vi "HomeVI.vi"() -> ()   [LabVIEW 2015]
uses:
  <vilib>/LabVIEW Interface for Arduino/Type Defs/Board Type.ctl
  <vilib>/express/express arith-compare/Formula/XNode/ExpressFormulaBlockNode.xnode
  <vilib>/LabVIEW Interface for Arduino/LabVIEW Interface for Arduino.lvlib
panel:
  in  "Tab Control":T1(tab)
  in  "Recipient's Name":string="DDU Smart Home"
  in  "Recipient's Email Address":string="ddusmarthome@gmail.com"
  in  "Arduino Mega COM Port":refnum<visa-resource-name>
  out "H_Current Mode":string
  in  "H_Mode Selector":enum32{"Automatic", "Manual"}(radio)
  in  "H_Light - Left":bool
  in  "H_Light - Right":bool
  in  "H_Fan Speed Regulator (% Percentage)":dbl(knob) scale=0.0..100.0
  out "H_Fan Speed ( % Percentage)":dbl(knob) scale=0.0..100.0
  out "H_Light - Left":bool
  out "H_Light - Right":bool
  out "H_Room Temprature":dbl(knob) scale=0.0..100.0
  out "H_Time":string
  out "K_Smoke":bool
  out "K_Light":bool
  in  "K_Mode Selector":enum32{"Automatic", "Manual"}(radio)
  out "K_Current Mode":string
  in  "K_Buzzer":bool
  in  "K_Light":bool
  out "K_Time":string
  out "B_Light":bool
  in  "B_Mode Selector":enum32{"Automatic", "Manual"}(radio)
  out "B_Current Mode":string
  in  "B_Light":bool
  out "B_Time":string
  in  "W_Light":bool
  out "W_Current Mode":string
  in  "W_Mode Selector":enum32{"Automatic", "Manual"}(radio)
  out "W_Light":bool
  out "W_Shower_Indicator":bool
  in  "Stop Button":bool
  in  "W_Mode Selector":enum32{"Automatic", "Manual"}(radio)
  out "W_Current Mode":string
  in  "W_Shower Switch":bool
  out "W_Time":string
  out "Last Intruder's Image":T2(plugin-control)
  # "Project Created By : \n                                     Patel Parth J. ( IC - 46 )\n                                     Patel Sarav M. (IC - 47)\n                                     Rai Aakash V. ( IC - 49 ) \n                                     Rupapara Pritesh N. ( IC - 51 )\n                                     Shah Vivek K. ( IC - 57 )"
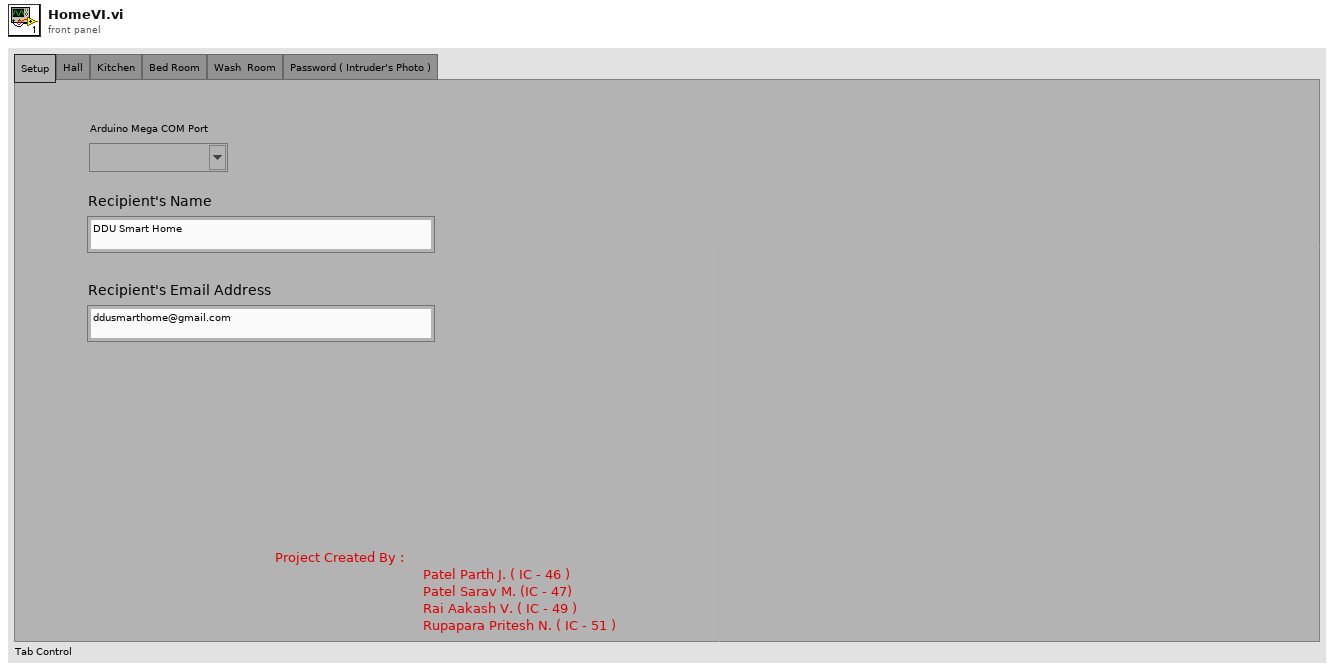
[diagram p1: front panel]
types:
  T1 = enum32{"Setup", "Hall", "Kitchen", "Bed Room", "Wash  Room", "Password ( Intruder's Photo )"}
  T2 = typedef "IMAQ Image.ctl" = refnum<image>
  T3 = typedef "LabVIEW Interface for Arduino.lvlib/Board Type.ctl" = enum16{"Uno", "Dimuelanove w/Atmega 328", "Mega 2560"}
  T4 = typedef "LabVIEW Interface for Arduino.lvlib/Arduino Resource.ctl" = cluster{"VISA resource":refnum<visa-resource-name>, "Board Type":T3, "Connection Type":enum8{"USB / Serial"}, "Bytes Per Packet (15)":u8}
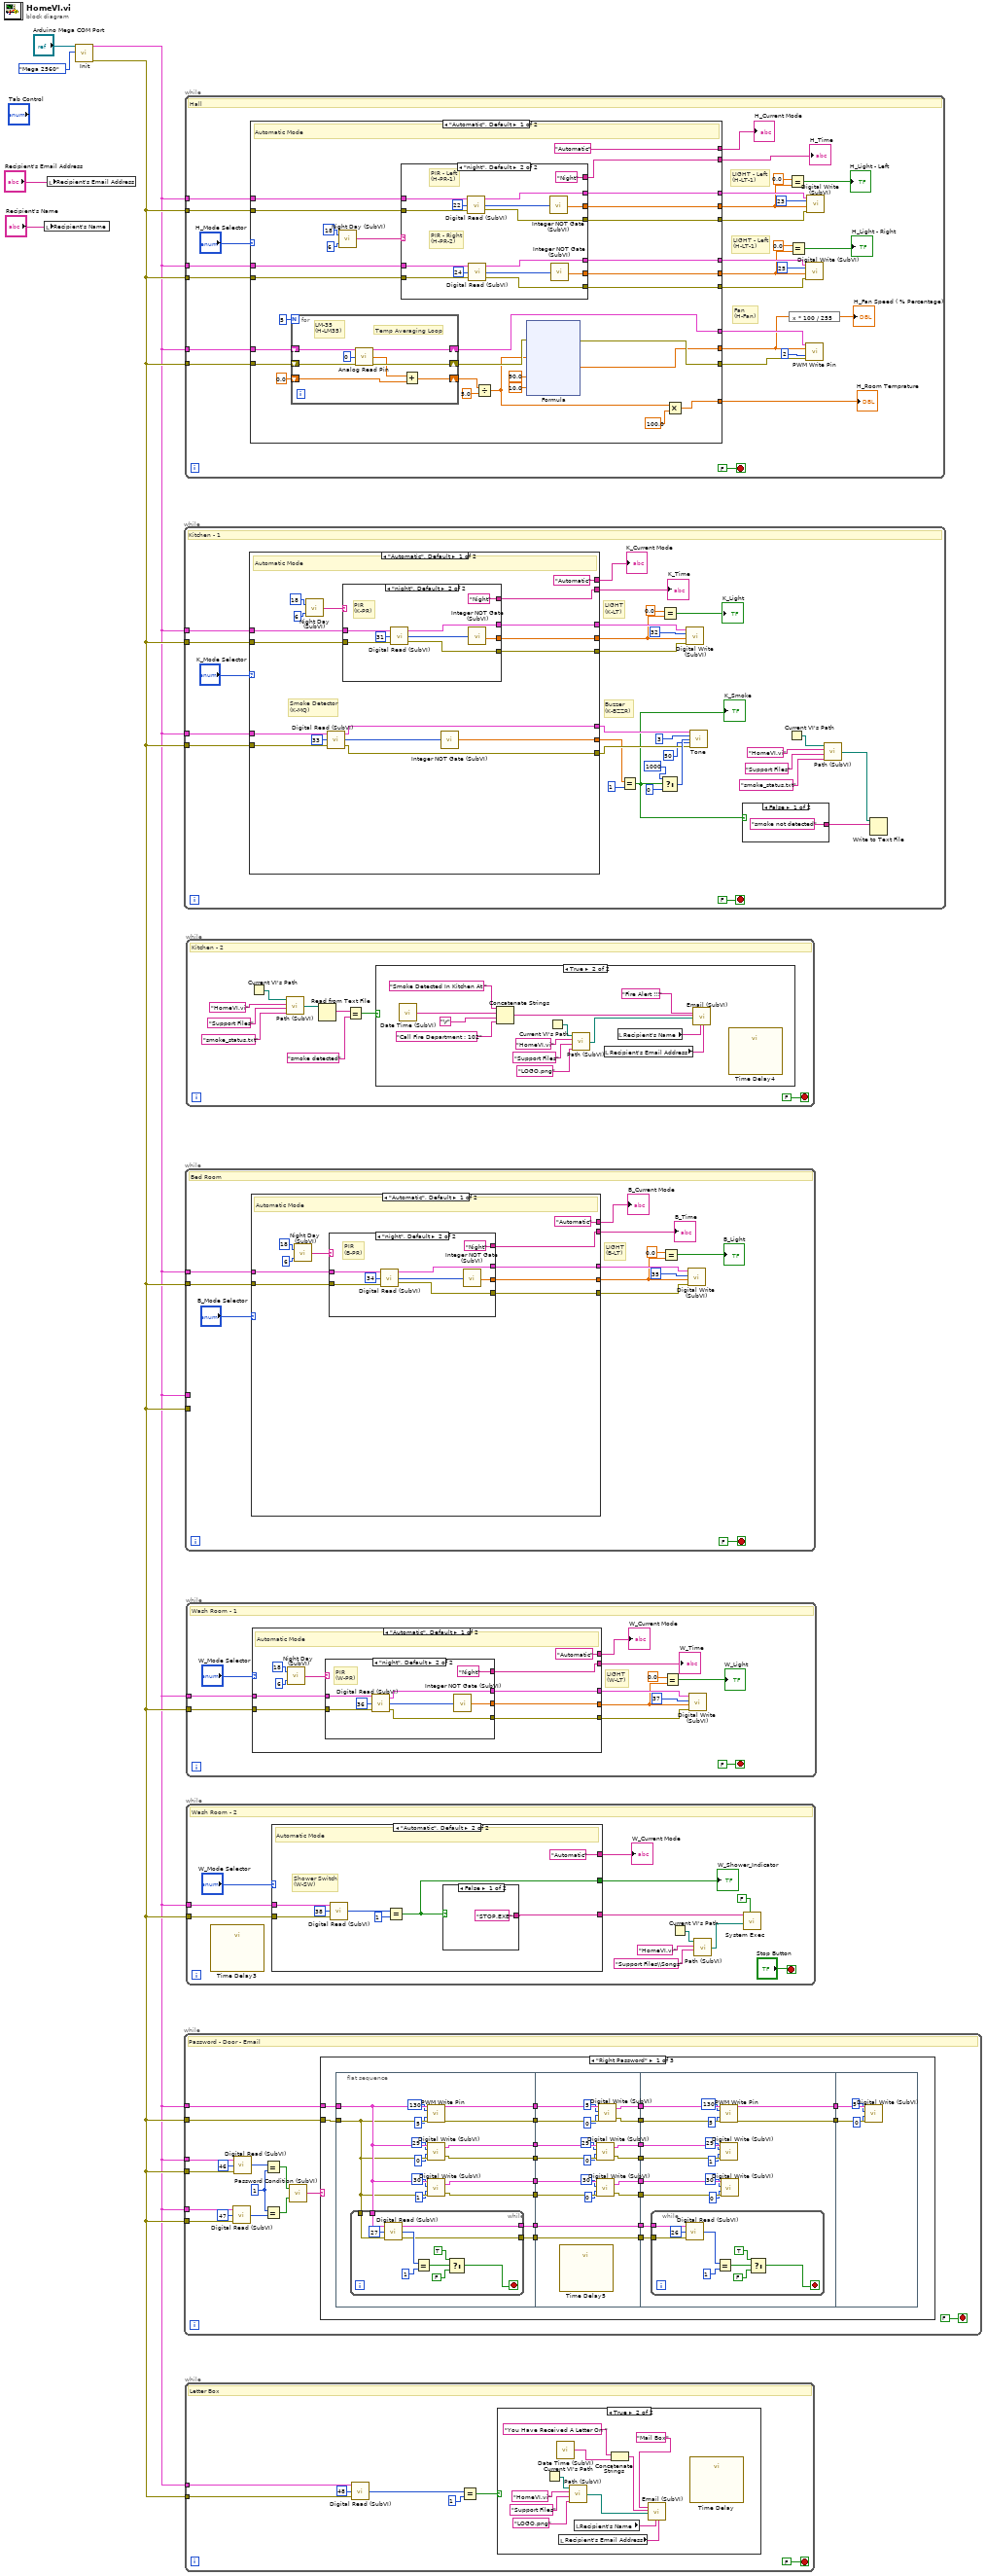
[diagram p0: block diagram]
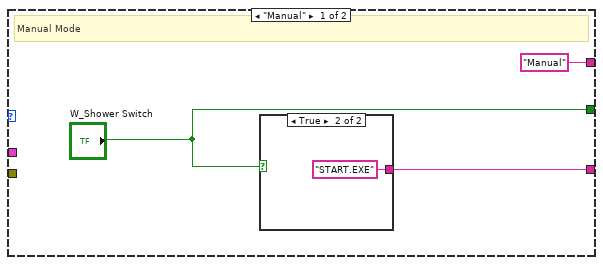
[diagram p4: hidden frame]
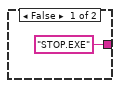
[diagram p5: hidden frame]
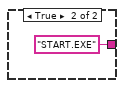
[diagram p6: hidden frame]
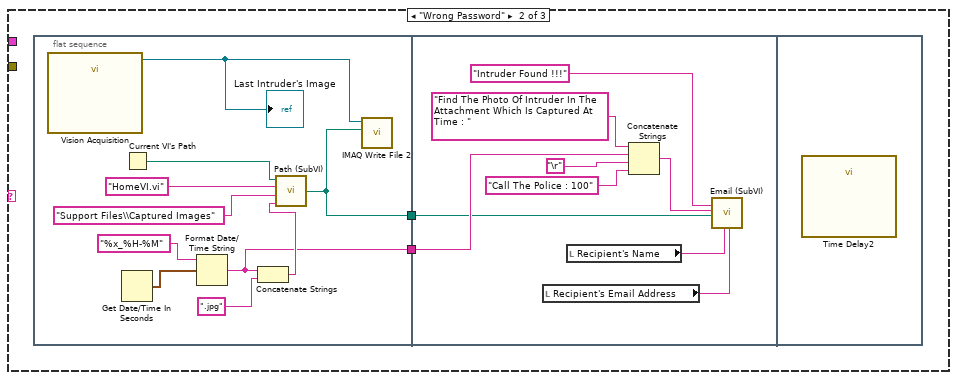
[diagram p7: hidden frame]
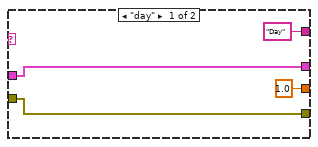
[diagram p9: hidden frame]
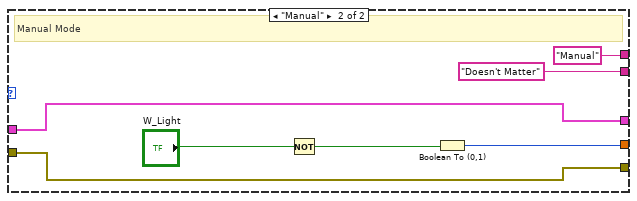
[diagram p10: hidden frame]
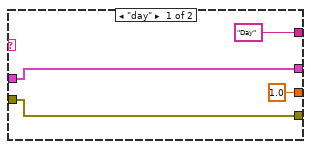
[diagram p11: hidden frame]
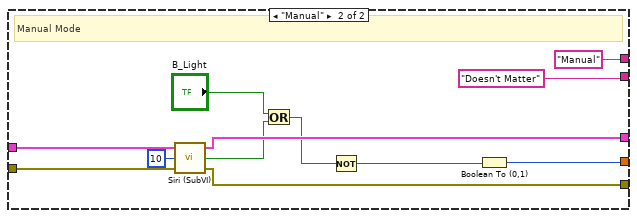
[diagram p12: hidden frame]
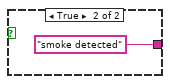
[diagram p13: hidden frame]
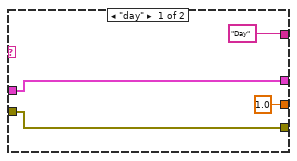
[diagram p14: hidden frame]
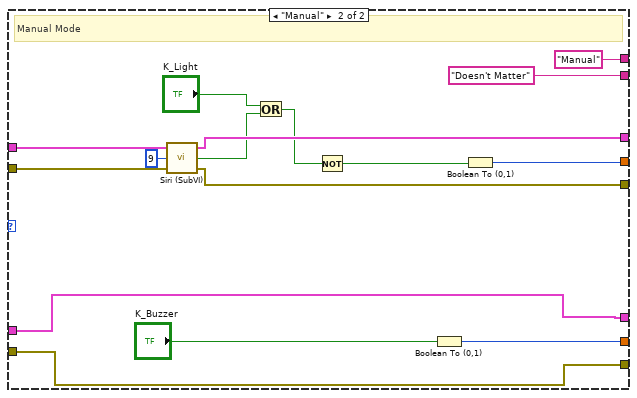
[diagram p15: hidden frame]
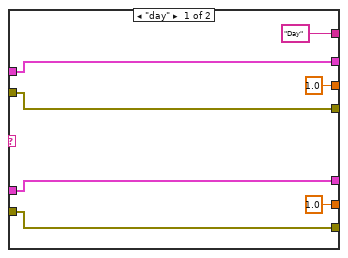
[diagram p16: hidden frame]
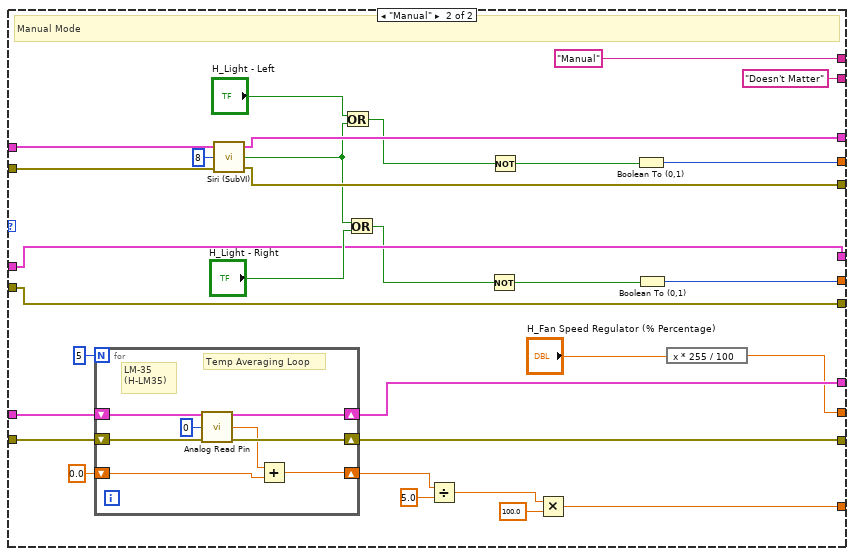
[diagram p17: hidden frame]
diagram:
  n1 = local write "Recipient's Name"("Recipient's Name") -> ()
  n2 = local write "Recipient's Email Address"("Recipient's Email Address") -> ()
  n3 = call <vilib>:"Init.vi"("VISA resource"="Arduino Mega COM Port", "Board Type (Uno)"=Board_Type."Mega 2560") -> ("Arduino Resource"=w4:T4, "error out"=w5:errorcluster)  [unwired: 16 in]
  n4 = while {
    tunnel: w4 -> [w29]
    tunnel: w5 -> [w28]
    tunnel: w4 -> [w20]
    tunnel: w5 -> [w19]
    stop <- FALSE stop-if-true
    # "Buzzer\n(K-BZZR)"
    # "LIGHT\n(K-LT)"
    # "Kitchen - 1"
    n5 = case shown="\"Automatic\", Default" "K_Mode Selector" {
      tunnel: ["Automatic" ("Current Mode") "Manual" ("Current Mode")] -> w35
      tunnel: [w54 w72] -> w34
      tunnel: [w53 w73] -> w33
      tunnel: [w52 w82] -> w32
      tunnel: w29 -> [w51 w74]
      tunnel: w28 -> [w50 w75]
      tunnel: [w49 w77] -> w23
      tunnel: [w48 w78] -> w24
      tunnel: [w40 w80] -> w22
      tunnel: w20 -> [w47 w78]
      tunnel: w19 -> [w46 w77]
      tunnel: [w39 "Doesn't Matter" ("K_Time")] -> w7
      frame "Automatic", Default {
        # "Smoke Detector\n(K-MQ)"
        # "Automatic Mode"
        n6 = call "Night Day (SubVI).vi"("To This (24HR)"=6 ("To This (24 HR)"), "From This (24 HR)"=18 ("From This (24HR)")) -> ("Time (CurrentTime-B/W-Range?Night:Day)"=w42:string)
        n7 = call "Digital Read (SubVI).vi"("error in (no error)"=w46, "Digital Input Pin"=u8 33, "Arduino Resource in"=w47) -> ("error out"=w49:errorcluster, "Value"=w41:u8, "Arduino Resource out"=w48:T4)
        n8 = case shown="\"night\", Default" w42 {
          tunnel: [w59 w66] -> w54
          tunnel: [w58 w65] -> w53
          tunnel: [1.0 ("Output State (Integer)") w64] -> w52
          tunnel: w51 -> [w58 w63]
          tunnel: w50 -> [w59 w62]
          tunnel: ["Day" ("K_Time") "Night" ("K_Time")] -> w39
          frame "day" {
          }
          frame "night", Default {
            # "PIR\n(K-PR)"
            n9 = call "Digital Read (SubVI).vi"("error in (no error)"=w62, "Digital Input Pin"=u8 31, "Arduino Resource in"=w63) -> ("error out"=w66:errorcluster, "Value"=w67:u8, "Arduino Resource out"=w65:T4)
            n10 = call "Integer NOT Gate (SubVI).vi"("Input State(Integer)"=w67) -> ("Output State (Integer)"=w64:dbl)
          }
        }
        n11 = call "Integer NOT Gate (SubVI).vi"("Input State(Integer)"=w41) -> ("Output State (Integer)"=w40:dbl)
      }
      frame "Manual" {
        # "Manual Mode"
        n12 = call "Siri (SubVI).vi"("error in (no error)"=w75, "Voice Controlled Input Pin"=u8 9, "Arduino Resource in"=w74) -> ("error out"=w72:errorcluster, "Voice Command Status"=w68:bool, "Arduino Resource out"=w73:T4)
        n13 = Or(x="K_Light", y=w68) -> (x .or. y?=w70:bool)
        n14 = Not(x=w70) -> (.not. x?=w83:bool)
        n15 = Boolean To (0,1)(Boolean="K_Buzzer") -> (0, 1=w80:i16)
        n16 = Boolean To (0,1)(Boolean=w83) -> (0, 1=w82:i16)
      }
    }
    "K_Current Mode" <- w35
    "K_Time" <- w7
    n17 = Equal?(x=w22, y=u8 1) -> (x = y?=w14:bool)
    "K_Smoke" <- w14
    n18 = Select(t=1000, s=w14, f=0) -> (s? t:f=w25:i32)
    n19 = Equal?(x=0.0, y=w32) -> (x = y?=→"K_Light":bool)
    n20 = call "Digital Write (SubVI).vi"("error in (no error)"=w34, "Value (0)"=w32, "Digital Output Pin"=u8 32, "Arduino Resource in"=w33) -> ()  [unwired: 2 out]
    n21 = call <vilib>:"Tone.vi"("Arduino Resource"=w24, "Tone DO Pin"=u8 3, "Frequency (0 Hz)"=w25, "Duration (1 ms)"=u32 50, "error in"=w23) -> ()  [unwired: 9 in, 2 out]
    n22 = case shown="False" w14 {
      tunnel: ["smoke not detected" ("text") "smoke detected" ("text")] -> w13
      frame False {
      }
      frame True {
      }
    }
    n23 = Current VI's Path() -> (path=w12:path)
    n24 = call "Path (SubVI).vi"("File Name"="smoke_status.txt", "Directory Name"="Support Files", "Current VI Name (Case Sensitive)"="HomeVI.vi", "Current VI Path"=w12) -> ("Path"=w8:path)
    n25 = Write to Text File(file (use dialog)=w8, text=w13) -> ()  [unwired: 2 in, 3 out]
  }
  n26 = while {
    tunnel: w4 -> [w96]
    tunnel: w5 -> [w97]
    tunnel: w4 -> [w94]
    tunnel: w5 -> [w95]
    tunnel: w4 -> [w85]
    tunnel: w5 -> [w84]
    stop <- FALSE stop-if-true
    w90 = u8 1 ("y")
    # "Password - Door - Email"
    n27 = call "Digital Read (SubVI).vi"("error in (no error)"=w95, "Digital Input Pin"=u8 47, "Arduino Resource in"=w94) -> ("Value"=w89:u8)  [unwired: 2 out]
    n28 = call "Digital Read (SubVI).vi"("error in (no error)"=w97, "Digital Input Pin"=u8 46, "Arduino Resource in"=w96) -> ("Value"=w91:u8)  [unwired: 2 out]
    n29 = Equal?(x=w91, y=w90) -> (x = y?=w87:bool)
    n30 = Equal?(x=w90, y=w89) -> (x = y?=w88:bool)
    n31 = call "Password Condition (SubVI).vi"("Y"=w88, "X"=w87) -> ("Password Condition"=w86:string)
    n32 = case shown="\"Right Password\"" w86 {
      tunnel: w85 -> [w102 _ _]
      tunnel: w84 -> [w101 _ _]
      frame "Right Password" {
        n33 = flat-sequence {
          tunnel: w102 -> [w134]
          tunnel: w101 -> [w133]
          tunnel: [w132] -> w118
          tunnel: [w131] -> w117
          tunnel: [w130] -> w116
          tunnel: [w129] -> w115
          tunnel: [w128] -> w114
          tunnel: [w127] -> w113
          tunnel: [w126] -> w112
          tunnel: [w125] -> w111
          tunnel: w118 -> [w151]
          tunnel: w117 -> [w150]
          tunnel: w116 -> [w165]
          tunnel: w115 -> [w164]
          tunnel: w114 -> [w163]
          tunnel: w113 -> [w162]
          tunnel: [w161] -> w110
          tunnel: [w160] -> w109
          tunnel: [w159] -> w108
          tunnel: [w158] -> w107
          tunnel: [w147] -> w106
          tunnel: [w146] -> w105
          tunnel: [w157] -> w104
          tunnel: w112 -> [w157]
          tunnel: [w156] -> w103
          tunnel: w111 -> [w156]
          tunnel: w110 -> [w181]
          tunnel: w109 -> [w180]
          tunnel: w108 -> [w179]
          tunnel: w107 -> [w178]
          tunnel: w106 -> [w177]
          tunnel: w105 -> [w176]
          tunnel: w104 -> [w175]
          tunnel: w103 -> [w174]
          tunnel: [w167] -> w100
          tunnel: [w166] -> w99
          tunnel: w100 -> [w194]
          tunnel: w99 -> [w193]
          frame #0 {
            n34 = while {
              tunnel: w134 -> [w140]
              tunnel: w133 -> [w139]
              tunnel: [w137] -> w126
              tunnel: [w136] -> w125
              stop <- w138 stop-if-true
              n35 = call "Digital Read (SubVI).vi"("error in (no error)"=w139, "Digital Input Pin"=u8 27, "Arduino Resource in"=w140) -> ("error out"=w136:errorcluster, "Value"=w145:u8, "Arduino Resource out"=w137:T4)
              n36 = Equal?(x=w145, y=u8 1) -> (x = y?=w143:bool)
              n37 = Select(t=TRUE, s=w143, f=FALSE) -> (s? t:f=w138:bool)
            }
            n38 = call <vilib>:"PWM Write Pin.vi"("Arduino Resource"=w134, "Duty Cycle (0 - 255)"=u8 130, "PWM Pin (3)"=u8 5, "error in"=w133) -> ("Arduino Resource"=w132:T4, "error out"=w131:errorcluster)  [unwired: 10 in]
            n39 = call "Digital Write (SubVI).vi"("error in (no error)"=w133, "Value (0)"=u8 0, "Digital Output Pin"=u8 29, "Arduino Resource in"=w134) -> ("error out"=w129:errorcluster, "Arduino Resource out"=w130:T4)
            n40 = call "Digital Write (SubVI).vi"("error in (no error)"=w133, "Value (0)"=u8 1, "Digital Output Pin"=u8 30, "Arduino Resource in"=w134) -> ("error out"=w127:errorcluster, "Arduino Resource out"=w128:T4)
          }
          frame #1 {
            n41 = call "Time Delay5"() -> ()  [unwired: 11 in, 1 out]
            n42 = call "Digital Write (SubVI).vi"("error in (no error)"=w164, "Value (0)"=u8 0, "Digital Output Pin"=u8 29, "Arduino Resource in"=w165) -> ("error out"=w160:errorcluster, "Arduino Resource out"=w161:T4)
            n43 = call "Digital Write (SubVI).vi"("error in (no error)"=w162, "Value (0)"=u8 0, "Digital Output Pin"=u8 30, "Arduino Resource in"=w163) -> ("error out"=w158:errorcluster, "Arduino Resource out"=w159:T4)
            n44 = call "Digital Write (SubVI).vi"("error in (no error)"=w150, "Value (0)"=u8 0 ("PWM Pin (3)"), "Digital Output Pin"=u8 5 ("Duty Cycle (0 - 255)"), "Arduino Resource in"=w151) -> ("error out"=w146:errorcluster, "Arduino Resource out"=w147:T4)
          }
          frame #2 {
            n45 = while {
              tunnel: w175 -> [w184]
              tunnel: w174 -> [w183]
              stop <- w185 stop-if-true
              n46 = call "Digital Read (SubVI).vi"("error in (no error)"=w183, "Digital Input Pin"=u8 26, "Arduino Resource in"=w184) -> ("Value"=w190:u8)  [unwired: 2 out]
              n47 = Equal?(x=w190, y=u8 1) -> (x = y?=w188:bool)
              n48 = Select(t=TRUE, s=w188, f=FALSE) -> (s? t:f=w185:bool)
            }
            n49 = call <vilib>:"PWM Write Pin.vi"("Arduino Resource"=w177, "Duty Cycle (0 - 255)"=u8 130, "PWM Pin (3)"=u8 5, "error in"=w176) -> ("Arduino Resource"=w167:T4, "error out"=w166:errorcluster)  [unwired: 10 in]
            n50 = call "Digital Write (SubVI).vi"("error in (no error)"=w180, "Value (0)"=u8 1, "Digital Output Pin"=u8 29, "Arduino Resource in"=w181) -> ()  [unwired: 2 out]
            n51 = call "Digital Write (SubVI).vi"("error in (no error)"=w178, "Value (0)"=u8 0, "Digital Output Pin"=u8 30, "Arduino Resource in"=w179) -> ()  [unwired: 2 out]
          }
          frame #3 {
            n52 = call "Digital Write (SubVI).vi"("error in (no error)"=w193, "Value (0)"=u8 0, "Digital Output Pin"=u8 5, "Arduino Resource in"=w194) -> ()  [unwired: 2 out]
          }
        }
      }
      frame "Wrong Password" {
        n53 = flat-sequence {
          tunnel: [w198] -> w196
          tunnel: [w197] -> w195
          tunnel: w196 -> [w213]
          tunnel: w195 -> [w211]
          frame #0 {
            n54 = call "Vision Acquisition"() -> ("Image Out"=w199:T2)  [unwired: 26 in, 1 out]
            "Last Intruder's Image" <- w199
            n55 = Get Date/Time In Seconds() -> (seconds since 1Jan1904=w205:timestamp)
            n56 = Current VI's Path() -> (path=w201:path)
            n57 = Format Date/Time String(time format string (%c)="%x_%H-%M", seconds (now)=w205) -> (date/time string=w198:string)  [unwired: 1 in]
            n58 = Concatenate Strings(w198, ".jpg" ("string")) -> (w200:string)
            n59 = call "Path (SubVI).vi"("File Name"=w200, "Directory Name"="Support Files\\Captured Images", "Current VI Name (Case Sensitive)"="HomeVI.vi", "Current VI Path"=w201) -> ("Path"=w197:path)
            n60 = call-poly "IMAQ Write File 2"("File Path"=w197, "Image"=w199) -> ()  [unwired: 8 in, 2 out]
          }
          frame #1 {
            n61 = local read "Recipient's Email Address"() -> (w207:string)
            n62 = local read "Recipient's Name"() -> (w208:string)
            n63 = Concatenate Strings("Find The Photo Of Intruder In The Attachment Which Is Captured At Time : " ("Body"), w213, "\r", "Call The Police : 100" ("string")) -> (w212:string)
            n64 = call "Email (SubVI).vi"("Subject"="Intruder Found !!!", "Body"=w212, "Attachment Path"=w211, "Recipients Name"=w208, "Recipients address"=w207) -> ()  [unwired: 15 in]
          }
          frame #2 {
            n65 = call "Time Delay2"() -> ()  [unwired: 11 in, 1 out]
          }
        }
      }
      frame "Normal Condition", Default {
        # "DO NOTHING"
      }
    }
  }
  n66 = while {
    tunnel: w4 -> [w227]
    tunnel: w4 -> [w226]
    tunnel: w4 -> [w225]
    tunnel: w5 -> [w224]
    tunnel: w5 -> [w222]
    tunnel: w5 -> [w221]
    stop <- FALSE stop-if-true
    # "Fan\n(H-Fan)"
    # "LIGHT - Left\n(H-LT-1)"
    # "LIGHT - Left\n(H-LT-1)"
    # "Hall"
    n67 = case shown="\"Automatic\", Default" "H_Mode Selector" {
      tunnel: ["Automatic" ("Current Mode") "Manual" ("Current Mode")] -> w242
      tunnel: [w269 w325] -> w241
      tunnel: [w268 w326] -> w240
      tunnel: [w267 w318] -> w239
      tunnel: [w266 w317] -> w238
      tunnel: [w265 w344] -> w229
      tunnel: [w264 w345] -> w233
      tunnel: [w261 w337] -> w237
      tunnel: [w263 w336] -> w236
      tunnel: [w262 w333] -> w234
      tunnel: w227 -> [w260 w328]
      tunnel: w226 -> [w259 w318]
      tunnel: w225 -> [w258 w341]
      tunnel: w224 -> [w257 w327]
      tunnel: w222 -> [w256 w317]
      tunnel: w221 -> [w255 w340]
      tunnel: [w253 w339] -> w220
      tunnel: [w244 "Doesn't Matter" ("Time")] -> w216
      frame "Automatic", Default {
        # "Automatic Mode"
        n68 = for {
          N: 5 -> [_]
          shift-right: [w302] -> w261
          shift-left: w258 -> [w301]
          shift-right: [w303] -> w272
          shift-left: w255 -> [w300]
          shift-right: [w298] -> w246
          shift-left: 0.0 -> [w296]
          # "Temp Averaging Loop"
          # "LM-35\n(H-LM35)"
          n69 = call <vilib>:"Analog Read Pin.vi"("Arduino Resource"=w301, "Analog Input Pin (0)"=u8 0, "error in"=w300) -> ("Arduino Resource"=w302:T4, "Voltage"=w297:dbl, "error out"=w303:errorcluster)  [unwired: 10 in]
          n70 = Add(x=w297, y=w296) -> (x+y=w298:dbl)
        }
        n71 = call "Night Day (SubVI).vi"("To This (24HR)"=6 ("To This (24 HR)"), "From This (24 HR)"=18 ("From This (24HR)")) -> ("Time (CurrentTime-B/W-Range?Night:Day)"=w250:string)
        n72 = case shown="\"night\", Default" w250 {
          tunnel: [w279 w293] -> w269
          tunnel: [w280 w292] -> w268
          tunnel: [w278 w291] -> w267
          tunnel: [w277 w290] -> w266
          tunnel: [1.0 ("Output State (Integer)") w289] -> w265
          tunnel: [1.0 ("Output State (Integer)") w288] -> w264
          tunnel: w260 -> [w280 w287]
          tunnel: w259 -> [w278 w286]
          tunnel: w257 -> [w279 w285]
          tunnel: w256 -> [w277 w284]
          tunnel: ["Day" ("Time") "Night" ("Time")] -> w244
          frame "day" {
          }
          frame "night", Default {
            # "PIR - Right\n(H-PR-2)"
            # "PIR - Left\n(H-PR-1)"
            n73 = call "Digital Read (SubVI).vi"("error in (no error)"=w285, "Digital Input Pin"=u8 22, "Arduino Resource in"=w287) -> ("error out"=w293:errorcluster, "Value"=w295:u8, "Arduino Resource out"=w292:T4)
            n74 = call "Digital Read (SubVI).vi"("error in (no error)"=w284, "Digital Input Pin"=u8 24, "Arduino Resource in"=w286) -> ("error out"=w290:errorcluster, "Value"=w294:u8, "Arduino Resource out"=w291:T4)
            n75 = call "Integer NOT Gate (SubVI).vi"("Input State(Integer)"=w295) -> ("Output State (Integer)"=w288:dbl)
            n76 = call "Integer NOT Gate (SubVI).vi"("Input State(Integer)"=w294) -> ("Output State (Integer)"=w289:dbl)
          }
        }
        n77 = Divide(x=w246, y=5.0) -> (x/y=w245:dbl)
        n78 = xnode ("Formula")("In_Voltage"=w245, "High_Temp"=90.0, "Low_Temp"=10.0, "error in (no error)"=w272) -> ("Result"=w262:dbl, "error out"=w263:errorcluster)
        n79 = Multiply(x=w245, y=100.0) -> (x*y=w253:dbl)
      }
      frame "Manual" {
        # "Manual Mode"
        n80 = for {
          N: 5 -> [_]
          shift-right: [w352] -> w337
          shift-left: w341 -> [w354]
          shift-right: [w350] -> w336
          shift-left: w340 -> [w353]
          shift-right: [w349] -> w331
          shift-left: 0.0 -> [w347]
          # "Temp Averaging Loop"
          # "LM-35\n(H-LM35)"
          n81 = call <vilib>:"Analog Read Pin.vi"("Arduino Resource"=w354, "Analog Input Pin (0)"=u8 0, "error in"=w353) -> ("Arduino Resource"=w352:T4, "Voltage"=w348:dbl, "error out"=w350:errorcluster)  [unwired: 10 in]
          n82 = Add(x=w348, y=w347) -> (x+y=w349:dbl)
        }
        n83 = call "Siri (SubVI).vi"("error in (no error)"=w327, "Voice Controlled Input Pin"=u8 8, "Arduino Resource in"=w328) -> ("error out"=w325:errorcluster, "Voice Command Status"=w320:bool, "Arduino Resource out"=w326:T4)
        n84 = Or(x="H_Light - Left", y=w320) -> (x .or. y?=w323:bool)
        n85 = Or(x=w320, y="H_Light - Right") -> (x .or. y?=w316:bool)
        n86 = Divide(x=w331, y=5.0) -> (x/y=w330:dbl)
        n87 = Not(x=w316) -> (.not. x?=w321:bool)
        n88 = Not(x=w323) -> (.not. x?=w346:bool)
        n89 = Multiply(x=w330, y=100.0) -> (x*y=w339:dbl)
        n90 = Boolean To (0,1)(Boolean=w346) -> (0, 1=w345:i16)
        n91 = Boolean To (0,1)(Boolean=w321) -> (0, 1=w344:i16)
        n92 = expression code="x * 255 / 100"("H_Fan Speed Regulator (% Percentage)") -> (w333:dbl)
      }
    }
    "H_Current Mode" <- w242
    "H_Room Temprature" <- w220
    "H_Time" <- w216
    n93 = Equal?(x=0.0, y=w233) -> (x = y?=→"H_Light - Left":bool)
    n94 = expression code="x * 100 / 255"(w234) -> (→"H_Fan Speed ( % Percentage)":dbl)
    n95 = Equal?(x=0.0, y=w229) -> (x = y?=→"H_Light - Right":bool)
    n96 = call "Digital Write (SubVI).vi"("error in (no error)"=w238, "Value (0)"=w229, "Digital Output Pin"=u8 25, "Arduino Resource in"=w239) -> ()  [unwired: 2 out]
    n97 = call <vilib>:"PWM Write Pin.vi"("Arduino Resource"=w237, "Duty Cycle (0 - 255)"=w234, "PWM Pin (3)"=u8 2, "error in"=w236) -> ()  [unwired: 10 in, 2 out]
    n98 = call "Digital Write (SubVI).vi"("error in (no error)"=w241, "Value (0)"=w233, "Digital Output Pin"=u8 23, "Arduino Resource in"=w240) -> ()  [unwired: 2 out]
  }
  n99 = while {
    tunnel: w4 -> [w356]
    tunnel: w5 -> [w355]
    stop <- FALSE stop-if-true
    # "Letter Box"
    n100 = call "Digital Read (SubVI).vi"("error in (no error)"=w355, "Digital Input Pin"=u8 48, "Arduino Resource in"=w356) -> ("Value"=w360:u8)  [unwired: 2 out]
    n101 = Equal?(x=w360, y=u8 1) -> (x = y?=w359:bool)
    n102 = case shown="True" w359 {
      frame False {
        # "DO NOTHING"
      }
      frame True {
        n103 = Current VI's Path() -> (path=w365:path)
        n104 = call "Date Time (SubVI).vi"() -> ("Date & Time"=w369:string)
        n105 = local read "Recipient's Email Address"() -> (w362:string)
        n106 = call "Path (SubVI).vi"("File Name"="LOGO.png" ("Directory Name"), "Directory Name"="Support Files", "Current VI Name (Case Sensitive)"="HomeVI.vi", "Current VI Path"=w365) -> ("Path"=w364:path)
        n107 = local read "Recipient's Name"() -> (w363:string)
        n108 = Concatenate Strings("You Have Received A Letter On " ("string"), w369) -> (w372:string)
        n109 = call "Email (SubVI).vi"("Subject"="Mail Box", "Body"=w372, "Attachment Path"=w364, "Recipients Name"=w363, "Recipients address"=w362) -> ()  [unwired: 15 in]
        n110 = call "Time Delay"() -> ()  [unwired: 11 in, 1 out]
      }
    }
  }
  n111 = while {
    tunnel: w4 -> [w377]
    tunnel: w5 -> [w376]
    tunnel: w5 -> [_]
    tunnel: w4 -> [_]
    stop <- FALSE stop-if-true
    # "LIGHT\n(B-LT)"
    # "Bed Room"
    n112 = case shown="\"Automatic\", Default" "B_Mode Selector" {
      tunnel: ["Automatic" ("Current Mode") "Manual" ("Current Mode")] -> w383
      tunnel: [w393 w411] -> w382
      tunnel: [w392 w412] -> w381
      tunnel: [w391 w417] -> w380
      tunnel: w377 -> [w390 w414]
      tunnel: w376 -> [w389 w413]
      tunnel: [w385 "Doesn't Matter" ("B_Time")] -> w373
      frame "Automatic", Default {
        # "Automatic Mode"
        n113 = call "Night Day (SubVI).vi"("To This (24HR)"=6 ("To This (24 HR)"), "From This (24 HR)"=18 ("From This (24HR)")) -> ("Time (CurrentTime-B/W-Range?Night:Day)"=w386:string)
        n114 = case shown="\"night\", Default" w386 {
          tunnel: [w397 w405] -> w393
          tunnel: [w398 w404] -> w392
          tunnel: [1.0 ("Output State (Integer)") w403] -> w391
          tunnel: w390 -> [w398 w402]
          tunnel: w389 -> [w397 w401]
          tunnel: ["Day" ("B_Time") "Night" ("B_Time")] -> w385
          frame "day" {
          }
          frame "night", Default {
            # "PIR\n(B-PR)"
            n115 = call "Digital Read (SubVI).vi"("error in (no error)"=w401, "Digital Input Pin"=u8 34, "Arduino Resource in"=w402) -> ("error out"=w405:errorcluster, "Value"=w406:u8, "Arduino Resource out"=w404:T4)
            n116 = call "Integer NOT Gate (SubVI).vi"("Input State(Integer)"=w406) -> ("Output State (Integer)"=w403:dbl)
          }
        }
      }
      frame "Manual" {
        # "Manual Mode"
        n117 = call "Siri (SubVI).vi"("error in (no error)"=w413, "Voice Controlled Input Pin"=u8 10, "Arduino Resource in"=w414) -> ("error out"=w411:errorcluster, "Voice Command Status"=w409:bool, "Arduino Resource out"=w412:T4)
        n118 = Or(x="B_Light", y=w409) -> (x .or. y?=w408:bool)
        n119 = Not(x=w408) -> (.not. x?=w418:bool)
        n120 = Boolean To (0,1)(Boolean=w418) -> (0, 1=w417:i16)
      }
    }
    "B_Current Mode" <- w383
    "B_Time" <- w373
    n121 = Equal?(x=0.0, y=w380) -> (x = y?=→"B_Light":bool)
    n122 = call "Digital Write (SubVI).vi"("error in (no error)"=w382, "Value (0)"=w380, "Digital Output Pin"=u8 35, "Arduino Resource in"=w381) -> ()  [unwired: 2 out]
  }
  n123 = while {
    stop <- FALSE stop-if-true
    # "Kitchen - 2"
    n124 = Current VI's Path() -> (path=w424:path)
    n125 = call "Path (SubVI).vi"("File Name"="smoke_status.txt", "Directory Name"="Support Files", "Current VI Name (Case Sensitive)"="HomeVI.vi", "Current VI Path"=w424) -> ("Path"=w420:path)
    n126 = Read from Text File(file (use dialog)=w420) -> (text=w419:string)  [unwired: 3 in, 3 out]
    n127 = Equal?(x=w419, y="smoke detected") -> (x = y?=w425:bool)
    n128 = case shown="True" w425 {
      frame False {
        # "DO NOTHING"
      }
      frame True {
        n129 = call "Date Time (SubVI).vi"() -> ("Date & Time"=w439:string)
        n130 = Concatenate Strings("Smoke Detected In Kitchen At ", w439, "\r", "Call Fire Department : 102") -> (w436:string)
        n131 = Current VI's Path() -> (path=w434:path)
        n132 = call "Path (SubVI).vi"("File Name"="LOGO.png" ("Directory Name"), "Directory Name"="Support Files", "Current VI Name (Case Sensitive)"="HomeVI.vi", "Current VI Path"=w434) -> ("Path"=w430:path)
        n133 = local read "Recipient's Email Address"() -> (w428:string)
        n134 = local read "Recipient's Name"() -> (w429:string)
        n135 = call "Email (SubVI).vi"("Subject"="Fire Alert !!!", "Body"=w436, "Attachment Path"=w430, "Recipients Name"=w429, "Recipients address"=w428) -> ()  [unwired: 15 in]
        n136 = call "Time Delay4"() -> ()  [unwired: 11 in, 1 out]
      }
    }
  }
  n137 = while {
    tunnel: w4 -> [w443]
    tunnel: w5 -> [w442]
    stop <- FALSE stop-if-true
    # "LIGHT\n(W-LT)"
    # "Wash Room - 1"
    n138 = case shown="\"Automatic\", Default" "W_Mode Selector" {
      tunnel: ["Automatic" ("Current Mode") "Manual" ("Current Mode")] -> w451
      tunnel: [w459 w477] -> w450
      tunnel: [w458 w478] -> w449
      tunnel: [w460 w479] -> w448
      tunnel: w443 -> [w462 w478]
      tunnel: w442 -> [w461 w477]
      tunnel: [w453 "Doesn't Matter" ("W_Time")] -> w441
      frame "Automatic", Default {
        # "Automatic Mode"
        n139 = call "Night Day (SubVI).vi"("To This (24HR)"=6 ("To This (24 HR)"), "From This (24 HR)"=18 ("From This (24HR)")) -> ("Time (CurrentTime-B/W-Range?Night:Day)"=w455:string)
        n140 = case shown="\"night\", Default" w455 {
          tunnel: w462 -> [w466 w473]
          tunnel: w461 -> [w465 w472]
          tunnel: [1.0 ("Output State (Integer)") w470] -> w460
          tunnel: [w465 w469] -> w459
          tunnel: [w466 w468] -> w458
          tunnel: ["Day" ("W_Time") "Night" ("W_Time")] -> w453
          frame "day" {
          }
          frame "night", Default {
            # "PIR\n(W-PR)"
            n141 = call "Digital Read (SubVI).vi"("error in (no error)"=w472, "Digital Input Pin"=u8 36, "Arduino Resource in"=w473) -> ("error out"=w469:errorcluster, "Value"=w474:u8, "Arduino Resource out"=w468:T4)
            n142 = call "Integer NOT Gate (SubVI).vi"("Input State(Integer)"=w474) -> ("Output State (Integer)"=w470:dbl)
          }
        }
      }
      frame "Manual" {
        # "Manual Mode"
        n143 = Not(x="W_Light") -> (.not. x?=w481:bool)
        n144 = Boolean To (0,1)(Boolean=w481) -> (0, 1=w479:i16)
      }
    }
    "W_Current Mode" <- w451
    "W_Time" <- w441
    n145 = Equal?(x=0.0, y=w448) -> (x = y?=→"W_Light":bool)
    n146 = call "Digital Write (SubVI).vi"("error in (no error)"=w450, "Value (0)"=w448, "Digital Output Pin"=u8 37, "Arduino Resource in"=w449) -> ()  [unwired: 2 out]
  }
  n147 = while {
    tunnel: w5 -> [w493]
    tunnel: w4 -> [w492]
    stop <- "Stop Button" stop-if-true
    # "Wash Room - 2"
    n148 = call "Time Delay3"() -> ()  [unwired: 11 in, 1 out]
    n149 = case shown="\"Automatic\", Default" "W_Mode Selector" {
      tunnel: w493 -> [_ w504]
      tunnel: w492 -> [_ w503]
      tunnel: [w496 w501] -> w491
      tunnel: ["W_Shower Switch" w500] -> w490
      tunnel: ["Manual" "Automatic"] -> w488
      frame "Manual" {
        # "Manual Mode"
        n150 = case shown="True" "W_Shower Switch" {
          tunnel: ["STOP.EXE" ("command line") "START.EXE" ("command line")] -> w496
          frame False {
          }
          frame True {
          }
        }
      }
      frame "Automatic", Default {
        # "Shower Switch\n(W-SW)"
        # "Automatic Mode"
        n151 = call "Digital Read (SubVI).vi"("error in (no error)"=w504, "Digital Input Pin"=u8 38, "Arduino Resource in"=w503) -> ("Value"=w505:u8)  [unwired: 2 out]
        n152 = Equal?(x=w505, y=u8 1) -> (x = y?=w500:bool)
        n153 = case shown="False" w500 {
          tunnel: ["STOP.EXE" ("command line") "START.EXE" ("command line")] -> w501
          frame False {
          }
          frame True {
          }
        }
      }
    }
    "W_Current Mode" <- w488
    "W_Shower_Indicator" <- w490
    n154 = Current VI's Path() -> (path=w486:path)
    n155 = call "Path (SubVI).vi"("Directory Name"="Support Files\\Songs", "Current VI Name (Case Sensitive)"="HomeVI.vi", "Current VI Path"=w486) -> ("Path"=w482:path)  [unwired: 1 in]
    n156 = call <vilib>:"System Exec.vi"("wait until completion? (T)"=FALSE, "working directory"=w482, "command line"=w491) -> ()  [unwired: 5 in, 4 out]
  }
